vi "Read Post Build VI from VIPB.vi"(8 "error in":errorcluster, 10 "VIPB File Path":path) -> (0 "error out":errorcluster, 1 "appended path":path, 2 "Post-Build_VI":string)   [LabVIEW 2019, in "VIPM.lvlib"]
uses:
  VIPM.lvlib
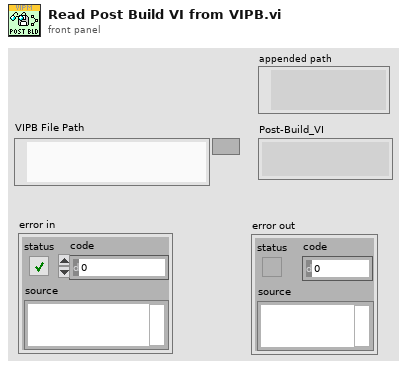
[diagram p1: front panel]
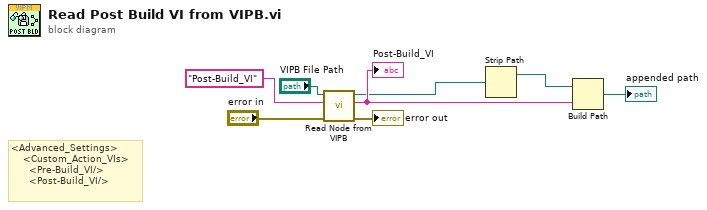
[diagram p0: block diagram]
diagram:
  # "<Advanced_Settings>\n    <Custom_Action_VIs>\n      <Pre-Build_VI/>\n      <Post-Build_VI/>"
  n1 = call "Read Node from VIPB.vi"("error in (no error)"="error in", "Node Name"="Post-Build_VI" ("XPath expression"), "VIPB File Path"="VIPB File Path") -> ("error out"=→"error out":errorcluster, "node text"=w3:string, "VIPB File Path out"=w2:path)  [unwired: 6 in]
  "Post-Build_VI" <- w3
  n2 = Strip Path(path=w2) -> (stripped path=w1:path)  [unwired: 1 out]
  n3 = Build Path(base path=w1, name or relative path=w3) -> (appended path=→"appended path":path)
